vi "Check.vi"(10 "Date":u8[](array[numeric])=[0, 0, 0, 0, 0, 0, 0] format="%x") -> (1 "Shift Data":u16, 2 "Msg Length":u16=7, 3 "Result":bool=TRUE)   [LabVIEW 2018]
uses:
  RFID GlobalVariable.vi
panel:
  out "_ByteCnt":u16=7
  # "Find first Character 'FF'"
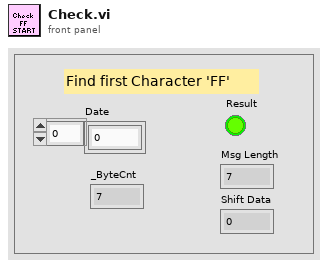
[diagram p1: front panel]
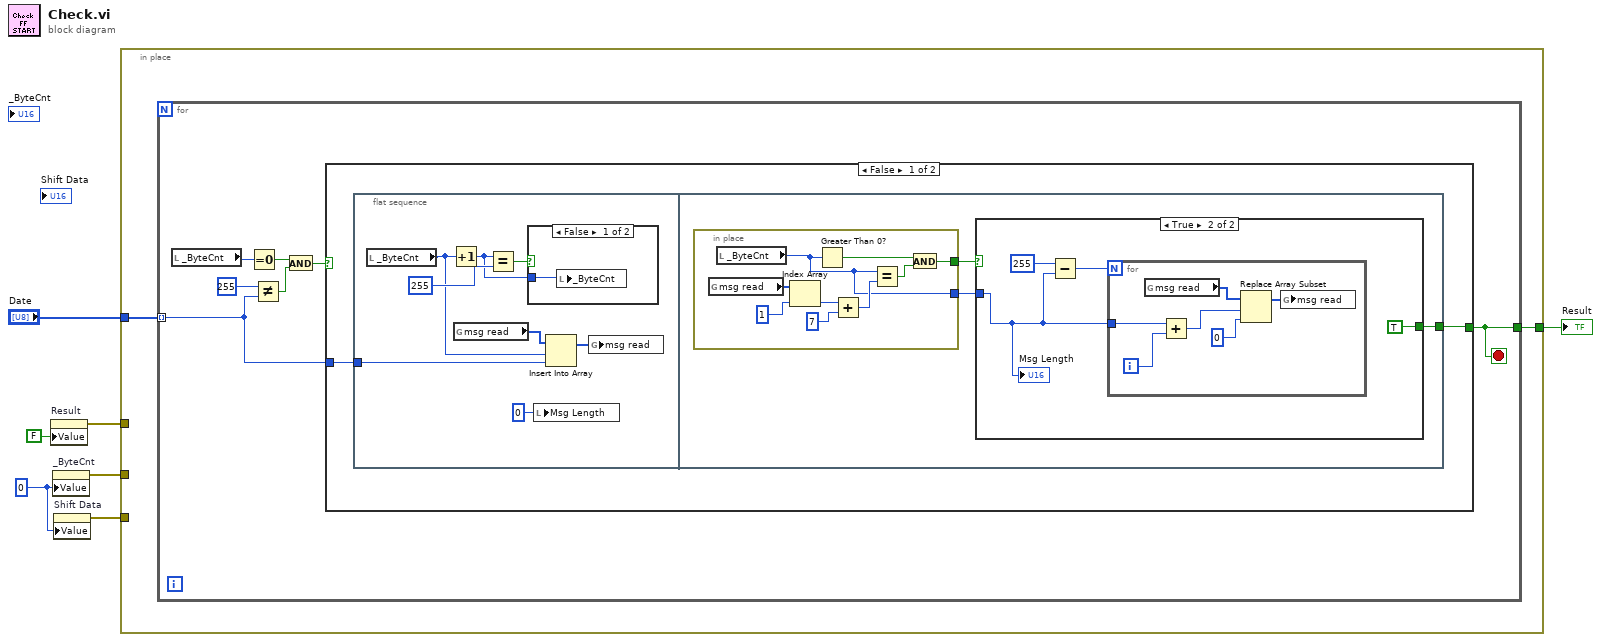
[diagram p0: block diagram]
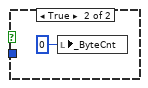
[diagram p2: hidden frame]
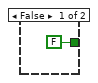
[diagram p3: hidden frame]
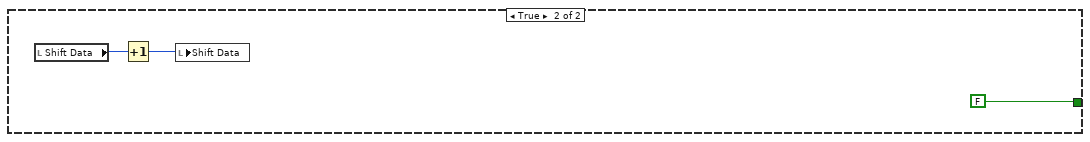
[diagram p4: hidden frame]
diagram:
  w1 = u16 0 ("_ByteCnt")
  n1 = property on="Result" class="Bool (strict)"("Value"=FALSE ("Result")) -> (error out=w7:errorcluster)  [unwired: 2 in, 1 out]
  n2 = property on="_ByteCnt" class="DigNum (strict)"("Value"=w1) -> (error out=w4:errorcluster)  [unwired: 2 in, 1 out]
  n3 = property on="Shift Data" class="DigNum (strict)"("Value"=w1) -> (error out=w2:errorcluster)  [unwired: 2 in, 1 out]
  n4 = in-place {
    in-place-border: w7 -> [_]
    in-place-border: "Date" -> [w9]
    in-place-border: w4 -> [_]
    in-place-border: [w8] -> w3
    in-place-border: w2 -> [_]
    n5 = for {
      tunnel: w9 -> [w15] mode=indexing
      tunnel: [w10] -> w8
      stop <- w10 stop-if-true
      n6 = local read "_ByteCnt"() -> (w11:u16)
      n7 = Equal To 0?(x=w11) -> (x = 0?=w13:bool)
      n8 = Not Equal?(x=u8 255, y=w15) -> (x != y?=w12:bool)
      n9 = And(x=w13, y=w12) -> (x .and. y?=w14:bool)
      n10 = case shown="False" w14 {
        tunnel: [w18 FALSE] -> w10
        tunnel: w15 -> [w17 _]
        frame False {
          n11 = flat-sequence {
            tunnel: w17 -> [w23]
            tunnel: [w29] -> w18
            frame #0 {
              n12 = local read "_ByteCnt"() -> (w20:u16)
              n13 = Increment(x=w20) -> (x+1=w24:u16)
              n14 = global read "RFID GlobalVariable.vi" "msg read"() -> (w21:u8[])
              n15 = Equal?(x=w24, y=255) -> (x = y?=w25:bool)
              n16 = case shown="False" w25 {
                tunnel: w24 -> [w27 _]
                frame False {
                  n17 = local write "_ByteCnt"(w27) -> ()
                }
                frame True {
                  n18 = local write "_ByteCnt"(u16 0 ("_head")) -> ()
                }
              }
              n19 = local write "Msg Length"(u16 0 ("Msg Length")) -> ()
              n20 = Insert Into Array(array=w21, index=w20, new element=w23) -> (w22:u8[])
              n21 = global write "RFID GlobalVariable.vi" "msg read"(w22) -> ()
            }
            frame #1 {
              n22 = in-place {
                in-place-border: [w34] -> w31
                in-place-border: [w32] -> w30
                n23 = global read "RFID GlobalVariable.vi" "msg read"() -> (w33:u8[])
                n24 = local read "_ByteCnt"() -> (w32:u16)
                n25 = Index Array(array=w33, index=1) -> (element=w38:u8)
                n26 = Greater Than 0?(x=w32) -> (x > 0?=w39:bool)
                n27 = Add(x=w38, y=7) -> (x+y=w35:i32)
                n28 = Equal?(x=w32, y=w35) -> (x = y?=w36:bool)
                n29 = And(x=w39, y=w36) -> (x .and. y?=w34:bool)
              }
              n30 = case shown="True" w31 {
                tunnel: w30 -> [_ w42]
                tunnel: [FALSE TRUE] -> w29
                frame False {
                }
                frame True {
                  n31 = Subtract(x=u16 255, y=w42) -> (x-y=w45:u16)
                  n32 = for {
                    N: w45 -> [_]
                    tunnel: w42 -> [w50]
                    i -> [w49]
                    n33 = global read "RFID GlobalVariable.vi" "msg read"() -> (w48:u8[])
                    n34 = Add(x=w50, y=w49) -> (x+y=w46:i32)
                    n35 = Replace Array Subset(array=w48, new element=u8 0 ("new element/subarray"), index=w46) -> (w47:u8[])
                    n36 = global write "RFID GlobalVariable.vi" "msg read"(w47) -> ()
                  }
                  "Msg Length" <- w42
                }
              }
            }
          }
        }
        frame True {
          n37 = local read "Shift Data"() -> (w53:u16)
          n38 = Increment(x=w53) -> (x+1=w52:u16)
          n39 = local write "Shift Data"(w52) -> ()
        }
      }
    }
  }
  "Result" <- w3
